vi "microphone.vi"() -> ()   [LabVIEW 2009]
uses:
  <vilib>/sound/lvsound.llb/Sound Format.ctl
  <vilib>/Analysis/baseanly.llb/Scale 1D.vi
  <vilib>/Analysis/NI_AALBase.lvlib
panel:
  out "error out":errorcluster
  in  "volume":dbl(slide) scale=10.0..32767.0
  out "Waveform Graph":dbl[](graph)
  in  "STOP":bool
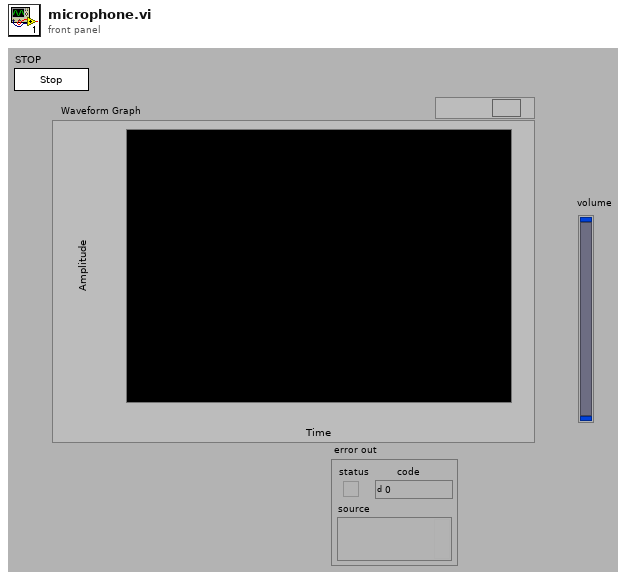
[diagram p1: front panel]
types:
  T1 = typedef "Sound Format.ctl" = cluster{"sound quality":enum16{"mono", "stereo"}, "rate":enum16{"11025", "22050", "44100", "8000"}, "bits per sample":enum16{"8 bit", "16 bit"}}
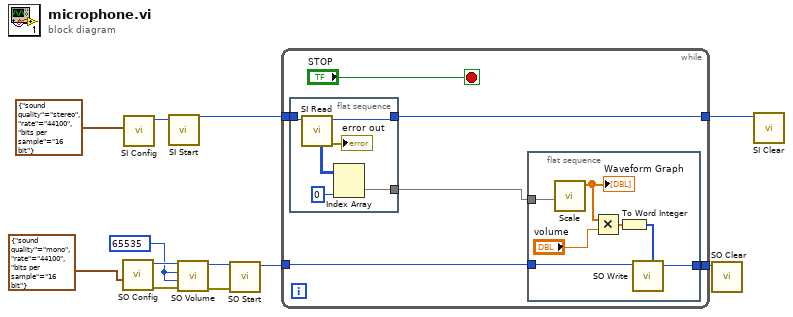
[diagram p0: block diagram]
diagram:
  w7 = u16 65535 ("left channel")
  n1 = call <vilib>:"SO Config.vi"("sound format"=T1 {"sound quality"=enum."mono", "rate"=enum."44100", "bits per sample"=enum."16 bit"}) -> ("error out"=w9:errorcluster, "task ID out"=w8:u32)  [unwired: 9 in]
  n2 = call <vilib>:"SI Config.vi"("sound format"=T1 {"sound quality"=enum."stereo", "rate"=enum."44100", "bits per sample"=enum."16 bit"}) -> ("task ID out"=w12:u32)  [unwired: 9 in, 1 out]
  n3 = call <vilib>:"SI Start.vi"("task ID in"=w12) -> ("task ID out"=w11:u32)  [unwired: 9 in, 1 out]
  n4 = call <vilib>:"SO Volume.vi"("error in (no error)"=w9, "right channel"=w7, "left channel"=w7, "task ID in"=w8) -> ("error out"=w4:errorcluster, "task ID out"=w3:u32)  [unwired: 6 in]
  n5 = call <vilib>:"SO Start.vi"("error in (no error)"=w4, "task ID in"=w3) -> ("task ID out"=w2:u32)  [unwired: 8 in, 1 out]
  n6 = while {
    tunnel: w11 -> [w17]
    tunnel: [w16] -> w10
    tunnel: w2 -> [w15]
    tunnel: [w14] -> w5
    stop <- "STOP" stop-if-true
    n7 = flat-sequence {
      tunnel: w17 -> [w24]
      tunnel: [w23] -> w16
      tunnel: [w20] -> w13
      frame #0 {
        n8 = call <vilib>:"SI Read.vi"("task ID in"=w24) -> ("error out"=→"error out":errorcluster, "task ID out"=w23:u32, "stereo 16-bit"=w21:i16[][])  [unwired: 5 in, 3 out]
        n9 = Index Array(array=w21, index (col)=0 ("disabled index (col)")) -> (element=w20:i16[])  [unwired: 1 in]
      }
    }
    n10 = flat-sequence {
      tunnel: w15 -> [w31]
      tunnel: [w30] -> w14
      tunnel: w13 -> [w25]
      frame #0 {
        n11 = call-poly <vilib>:"Scale.vi"("X"=w25) -> ("Y=(X-offset)/scale"=w26:dbl[])  [unwired: 3 out]
        "Waveform Graph" <- w26
        n12 = Multiply(x=w26, y="volume") -> (x*y=w28:dbl[])
        n13 = To Word Integer(number=w28) -> (16bit integer=w27:i16[])
        n14 = call <vilib>:"SO Write.vi"("mono 16-bit"=w27, "task ID in"=w31) -> ("task ID out"=w30:u32)  [unwired: 8 in, 1 out]
      }
    }
  }
  n15 = call <vilib>:"SO Clear.vi"("task ID in"=w5) -> ()  [unwired: 10 in, 1 out]
  n16 = call <vilib>:"SI Clear.vi"("task ID in"=w10) -> ()  [unwired: 10 in, 1 out]
